vi "HoldLevel.vi"(6 "Hold DC Offset":dbl=3.0, 9 "Hold Duration":dbl=8.0, 10 "SignalIn":dbl[](array[numeric]), 11 "Sample Rate":dbl) -> (3 "SignalOut":dbl[](array[numeric]))   [LabVIEW 2016]
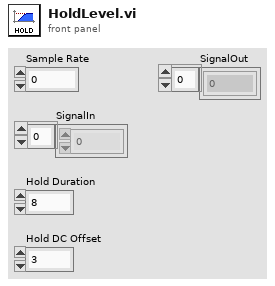
[diagram p1: front panel]
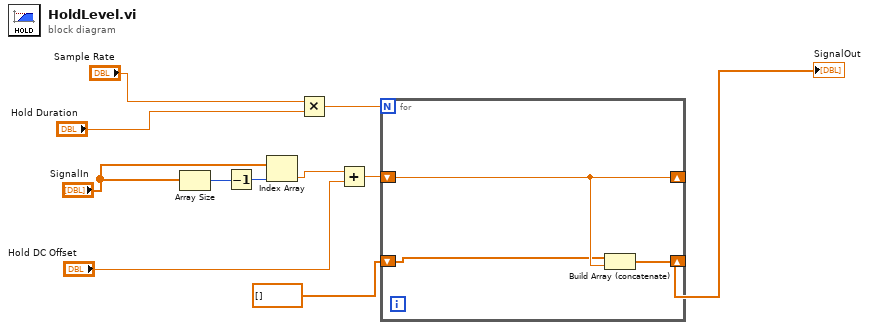
[diagram p0: block diagram]
diagram:
  n1 = Array Size(array="SignalIn") -> (size(s)=w9:i32)
  n2 = Decrement(x=w9) -> (x-1=w10:i32)
  n3 = Index Array(array="SignalIn", index=w10) -> (element=w2:dbl)
  n4 = Multiply(x="Sample Rate", y="Hold Duration") -> (x*y=w7:dbl)
  n5 = Add(x=w2, y="Hold DC Offset") -> (x+y=w3:dbl)
  n6 = for {
    N: w7 -> [_]
    shift-right: [w14] -> _
    shift-left: w3 -> [w14]
    shift-right: [w12] -> w8
    shift-left: dbl[] [] -> [w13]
    n7 = Build Array (concatenate)(w13, w14) -> (w12:dbl[])
  }
  "SignalOut" <- w8
